vi "Delete BrowerComponent.vi"(8 "error in (no error)":errorcluster, 10 "BrowerComponentID(\"\")":string, 11 "BrowerController in":refnum<class "BrowerController.lvclass">) -> (0 "error out":errorcluster, 3 "BrowerController out":refnum<class "BrowerController.lvclass">)   [LabVIEW 2015, in "BrowerController.lvclass"]
uses:
  BrowerController.lvclass
  BrowerController.lvclass/BrowerController.ctl
  Models/BrowerComponent/BrowerComponent/BrowerComponent.lvclass
  Models/BrowerTree/BrowerTree.lvclass
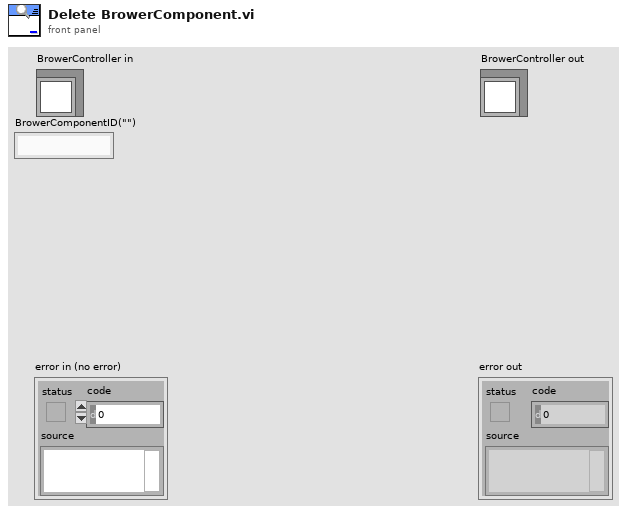
[diagram p1: front panel]
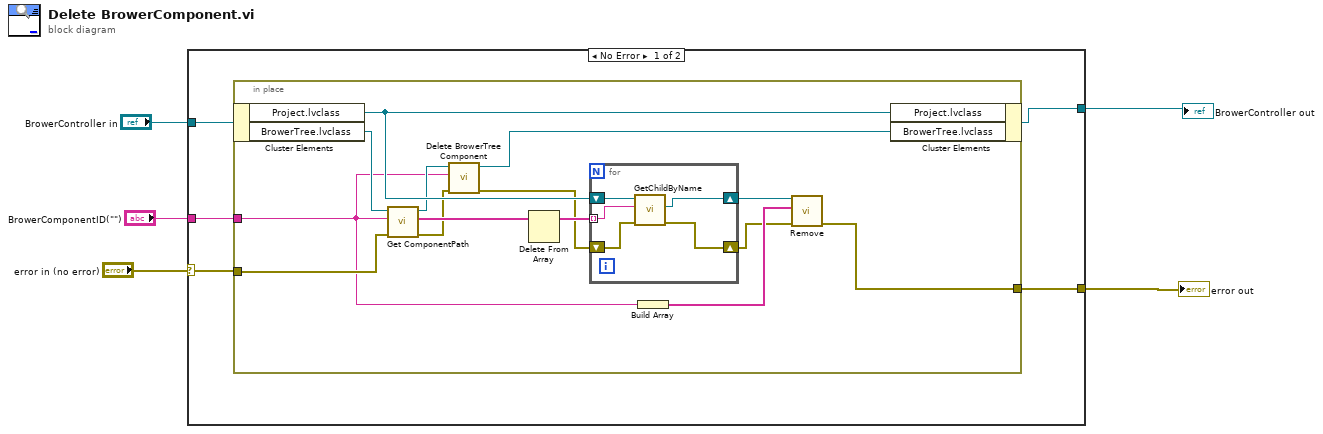
[diagram p0: block diagram]
diagram:
  n1 = case shown="No Error" "error in (no error)" {
    selector: "error in (no error)" -> [w10 w31]
    tunnel: [w6 w31] -> w4
    tunnel: [w8 w30] -> w3
    tunnel: "BrowerController in" -> [w9 w30]
    tunnel: "BrowerComponentID(\"\")" -> [w7 _]
    frame No Error {
      n2 = in-place {
        in-place-border: w10 -> [w16]
        in-place-border: w7 -> [w14]
        in-place-border: [w19] -> w6
        n3 = in-place-cluster #1(w9) -> ("Project.lvclass"=w18:refnum<class "BrowerComponent.lvclass">, "BrowerTree.lvclass"=w17:refnum<class "BrowerTree.lvclass">)
        n4 = call "Get ComponentPath.vi"("error in (no error)"=w16, "BrowerComponentID(\"\")"=w14, "BrowerTree in"=w17) -> ("error out"=w12:errorcluster, "Navigate Tree:Get Paths"=w24:string[], "BrowerTree out"=w15:refnum<class "BrowerTree.lvclass">)  [unwired: 6 in]
        n5 = call "Delete BrowerTree Component.vi"("error in (no error)"=w12, "BrowerComponentID(\"\")"=w14, "BrowerTree in"=w15) -> ("error out"=w11:errorcluster, "BrowerTree out"=w13:refnum<class "BrowerTree.lvclass">)  [unwired: 7 in]
        n6 = Delete From Array(array=w24) -> (array with subset deleted=w23:string[])  [unwired: 2 in, 1 out]
        n7 = for {
          tunnel: w23 -> [w28] mode=indexing
          shift-right: [w26] -> w22
          shift-left: w18 -> [w29]
          shift-right: [w25] -> w20
          shift-left: w11 -> [w27]
          n8 = call-dynamic "GetChildByName.vi"("error in (no error)"=w27, "BrowerComponentID(\"\")"=w28, "reference in"=w29) -> ("error out"=w25:errorcluster, "BrowerComponent"=w26:refnum<class "BrowerComponent.lvclass">)  [unwired: 6 in, 1 out]
        }
        n9 = Build Array(w14) -> (w21:string[])
        n10 = call-dynamic "Remove.vi"("error in (no error)"=w20, "BrowerComponentIDs(\"\")"=w21, "reference in"=w22) -> ("error out"=w19:errorcluster)  [unwired: 7 in, 1 out]
        n11 = in-place-cluster #1("Project.lvclass"=w18, "BrowerTree.lvclass"=w13) -> (w8:refnum<class "BrowerController.lvclass">)
      }
    }
    frame Error {
    }
  }
  "error out" <- w4
  "BrowerController out" <- w3
